vi "Write Assertion Type.vi"(10 "Assertion Type":T1=enum."Pass", 11 "Assertion Result In":refnum<class "Assertion Result.lvclass">) -> (3 "Assertion Result Out":refnum<class "Assertion Result.lvclass">)   [LabVIEW 2020, in "Assertion Result.lvclass"]
doc: "only writes type if it is not already set upstreams"
uses:
  Assertion Result.lvclass
  Public/TypeDefs/Assertion Type.ctl
  Assertion Result.lvclass/Assertion Result.ctl
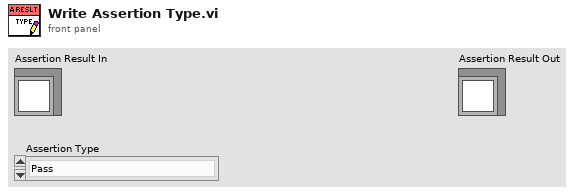
[diagram p1: front panel]
types:
  T1 = typedef "Assertion Result.lvclass/Assertion Type.ctl" = enum16{"None", "Pass", "Fail", "Skip", "Pass if Equal", "Fail if Equal", "Pass if Error", "Fail if Error", "Pass if", "Fail if"}
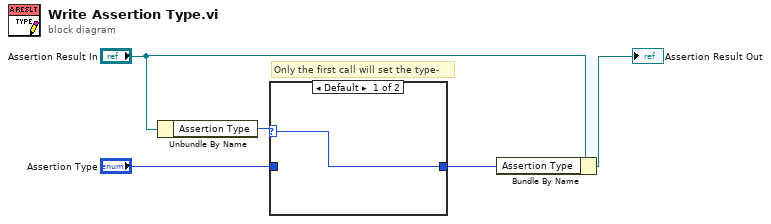
[diagram p0: block diagram]
diagram:
  # "Only the first call will set the type-"
  n1 = Unbundle By Name("Assertion Result In") -> ("Assertion Type"=w3:T1)
  n2 = case shown="Default" w3 {
    selector: w3 -> [w6 _]
    tunnel: "Assertion Type" -> [_ w7]
    tunnel: [w6 w7] -> w1
    frame Default {
    }
    frame "None" {
    }
  }
  n3 = Bundle By Name(cluster="Assertion Result In", "Assertion Type"=w1) -> (→"Assertion Result Out":refnum<class "Assertion Result.lvclass">)
